vi "Library Children Data.vi"(7 "Destination":path=path "", 8 "Error In":errorcluster, 11 "Library In":refnum<vi>) -> (0 "Error Out":errorcluster, 2 "Array":refnum<class "Map.lvclass">[](array[class]), 3 "Library Out":refnum<vi>)   [LabVIEW 2018, in "Scripts.lvlib"]
uses:
  Scripts.lvlib
  Toolkit/Data/Map/Map.lvclass
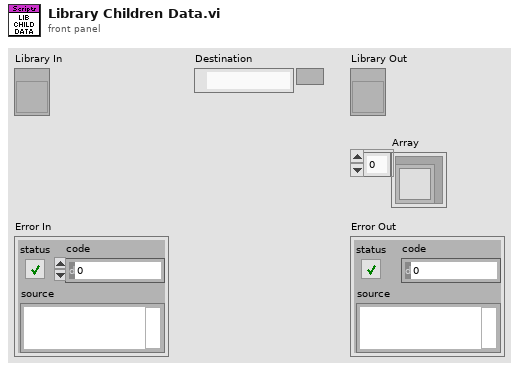
[diagram p1: front panel]
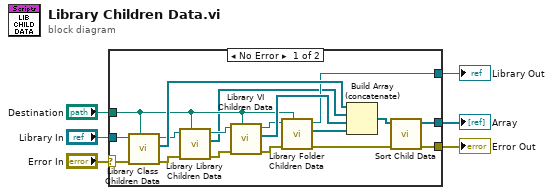
[diagram p0: block diagram]
diagram:
  n1 = case shown="No Error" "Error In" {
    selector: "Error In" -> [w24 w25]
    tunnel: [w18 _] -> w6
    tunnel: [w19 w25] -> w5
    tunnel: [w14 w26] -> w4
    tunnel: "Library In" -> [w23 w26]
    tunnel: "Destination" -> [w8 _]
    frame No Error {
      n2 = call "Library Class Children Data.vi"("Destination"=w8, "Error In"=w24, "Library In"=w23) -> ("Error Out"=w9:errorcluster, "Data"=w22:refnum<class "Map.lvclass">[], "Library Out"=w12:refnum<vi>)  [unwired: 6 in]
      n3 = call "Library Library Children Data.vi"("Destination"=w8, "Error In"=w9, "Library In"=w12) -> ("Error Out"=w10:errorcluster, "Data"=w7:refnum<class "Map.lvclass">[], "Library Out"=w11:refnum<vi>)  [unwired: 6 in]
      n4 = call "Library VI Children Data.vi"("Destination"=w8, "Error In"=w10, "Library In"=w11) -> ("Error Out"=w17:errorcluster, "Data"=w21:refnum<class "Map.lvclass">[], "Library Out"=w15:refnum<vi>)  [unwired: 6 in]
      n5 = call "Library Folder Children Data.vi"("Destination"=w8, "Error In"=w17, "Library In"=w15) -> ("Error Out"=w16:errorcluster, "Data"=w13:refnum<class "Map.lvclass">[], "Library Out"=w14:refnum<vi>)  [unwired: 6 in]
      n6 = Build Array (concatenate)(w22, w7, w21, w13) -> (w20:refnum<class "Map.lvclass">[])
      n7 = call "Sort Child Data.vi"("Error In"=w16, "Unsorted In"=w20) -> ("Error Out"=w19:errorcluster, "Sorted Out"=w18:refnum<class "Map.lvclass">[])  [unwired: 8 in]
    }
    frame Error {
    }
  }
  "Array" <- w6
  "Error Out" <- w5
  "Library Out" <- w4
